vi "Get VI Metrics(冲突时的文件备份2013-05-03 10-41-32).vi"() -> ()   [LabVIEW 2012]
panel:
  in  "停止按钮":bool
  out "VI Metrics":T1
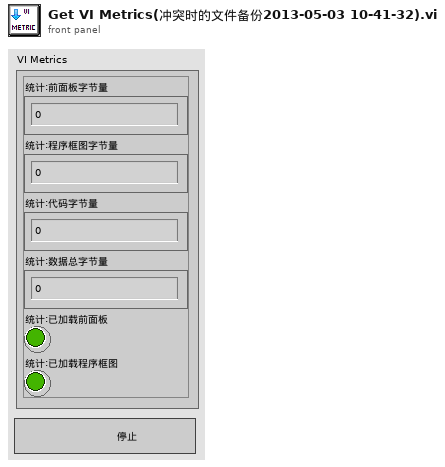
[diagram p1: front panel]
types:
  T1 = cluster{"统计:前面板字节量":u32, "统计:程序框图字节量":u32, "统计:代码字节量":u32, "统计:数据总字节量":u32, "统计:已加载前面板":bool, "统计:已加载程序框图":bool}
  T2 = cluster{"Metric.FPSize":u32, "Metric.BDSize":u32, "Metric.CodeSize":u32, "Metric.DataSize":u32, "PanelLoaded":bool, "DiagramLoaded":bool}
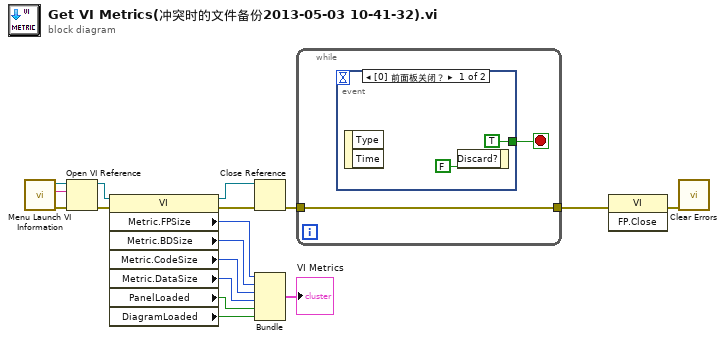
[diagram p0: block diagram]
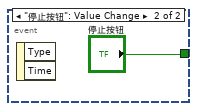
[diagram p2: hidden frame]
diagram:
  n1 = call <vilib>:"Menu Launch VI Information.vi"() -> ("error out"=w15:errorcluster, "Menu Launch:VI"=w17:string, "Menu Launch:App"=w16:refnum<vi>)  [unwired: 9 in]
  n2 = Open VI Reference(application reference (local)=w16, vi path=w17, error in (no error)=w15) -> (vi reference=w14:refnum<vi>, error out=w13:errorcluster)  [unwired: 3 in]
  n3 = property class="VI"(reference=w14, error in=w13) -> (reference out=w11:refnum<vi>, error out=w12:errorcluster, "Metric.FPSize"=w9:u32, "Metric.BDSize"=w8:u32, "Metric.CodeSize"=w7:u32, "Metric.DataSize"=w6:u32, "PanelLoaded"=w5:bool, "DiagramLoaded"=w4:bool)
  n4 = Close Reference(reference=w11, error in (no error)=w12) -> (error out=w3:errorcluster)
  n5 = Bundle("Metric.FPSize"=w9, "Metric.BDSize"=w8, "Metric.CodeSize"=w7, "Metric.DataSize"=w6, "PanelLoaded"=w5, "DiagramLoaded"=w4) -> (→"VI Metrics":T2)  [unwired: 1 in]
  n6 = while {
    tunnel: w3 -> [w18]
    tunnel: [w18] -> w2
    stop <- w19 stop-if-true
    n7 = event shown="[0] 前面板关闭？" {
      selector: _ -> [_ _]
      dyn-events: _ -> [_ _]
      timeout: _ -> [_ _]
      tunnel: [TRUE ("停止按钮") "停止按钮"] -> w19
      event Panel Close? {
        n8 = event-data() -> ()  [unwired: 1 in, 2 out]
        n9 = event-data("Discard?"=FALSE ("放弃？")) -> ()  [unwired: 1 in, 1 out]
      }
      event "停止按钮": Value Change {
        n10 = event-data() -> ()  [unwired: 1 in, 2 out]
      }
    }
  }
  n11 = invoke class="VI" method="FP.Close"(error in=w2) -> (error out=w1:errorcluster)  [unwired: 2 in, 2 out]
  n12 = call <vilib>:"Clear Errors.vi"("error in (no error)"=w1) -> ()  [unwired: 6 in, 1 out]
